vi "Settings_page.vi"() -> (0 "STOP ALL OUT":bool)   [LabVIEW 2016]
panel:
  in  "STOP ALL":bool
  in  "Exit":bool
  in  "Critical Level Settings":bool
  in  "Serial Settings":bool
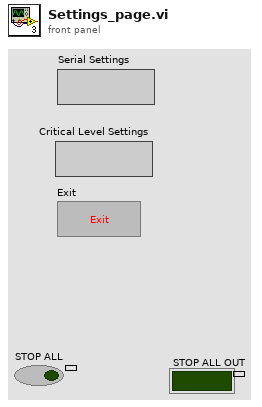
[diagram p1: front panel]
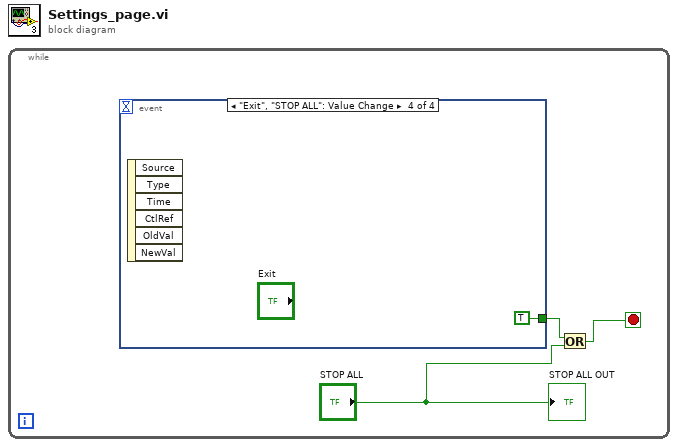
[diagram p0: block diagram]
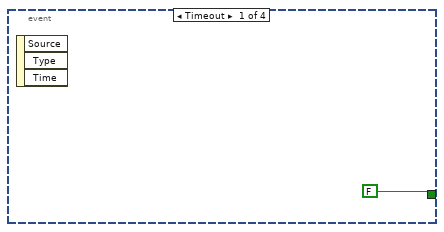
[diagram p2: hidden frame]
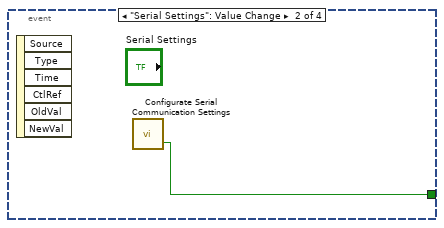
[diagram p3: hidden frame]
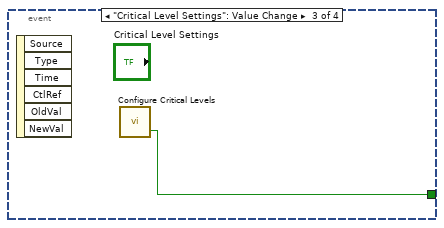
[diagram p4: hidden frame]
diagram:
  n1 = while {
    stop <- w2 stop-if-true
    n2 = event shown="[3] \"Exit\", \"STOP ALL\": Value Change" {
      selector: _ -> [_ _ _ _]
      dyn-events: _ -> [_ _ _ _]
      timeout: _ -> [_ _ _ _]
      tunnel: [FALSE w5 w6 TRUE ("STOP ALL OUT")] -> w3
      event Timeout {
        n3 = event-data() -> ()  [unwired: 1 in, 3 out]
      }
      event "Serial Settings": Value Change {
        n4 = event-data() -> ()  [unwired: 1 in, 6 out]
        n5 = call "Configurate Serial Communication Settings.vi"() -> ("STOP ALL 2"=w5:bool)  [unwired: 2 in, 1 out]
      }
      event "Critical Level Settings": Value Change {
        n6 = event-data() -> ()  [unwired: 1 in, 6 out]
        n7 = call "Configure Critical Levels.vi"() -> ("STOP ALL OUT"=w6:bool)  [unwired: 3 in]
      }
      event "Exit", "STOP ALL": Value Change {
        n8 = event-data() -> ()  [unwired: 1 in, 6 out]
      }
    }
    n9 = Or(x=w3, y="STOP ALL") -> (x .or. y?=w2:bool)
    "STOP ALL OUT" <- "STOP ALL"
  }
